vi "Subvi in range U16.vi"(8 "Max":u16, 9 "Input":u16, 10 "Min":u16) -> (1 "In range":bool)   [LabVIEW 2017]
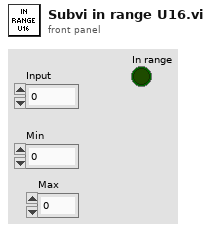
[diagram p1: front panel]
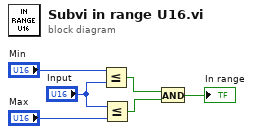
[diagram p0: block diagram]
diagram:
  n1 = Less Or Equal?(x="Min", y="Input") -> (x <= y?=w5:bool)
  n2 = Less Or Equal?(x="Input", y="Max") -> (x <= y?=w4:bool)
  n3 = And(x=w5, y=w4) -> (x .and. y?=→"In range":bool)
